vi "Get Function Status.vi"(8 "error in (no error)":errorcluster, 10 "Function.lvclass":refnum<class "Function.lvclass">, 11 "Results in":refnum<class "Results.lvclass">) -> (0 "error out":errorcluster, 3 "Results out":refnum<class "Results.lvclass">)   [LabVIEW 2016, in "Result Actor.lvlib" / "Results.lvclass"]
uses:
  <userlib>/Common Components/Results/Results.lvclass
  <userlib>/Common Components/Function Actor/Function.lvclass
  <userlib>/Common Components/Controller/Unique Function ID.ctl
  <userlib>/Common Components/Function Actor/Function.lvclass/Function.ctl
  <userlib>/Common Components/Results/Results.lvclass/Results.ctl
  <userlib>/Common Components/Controller/Controller.lvclass
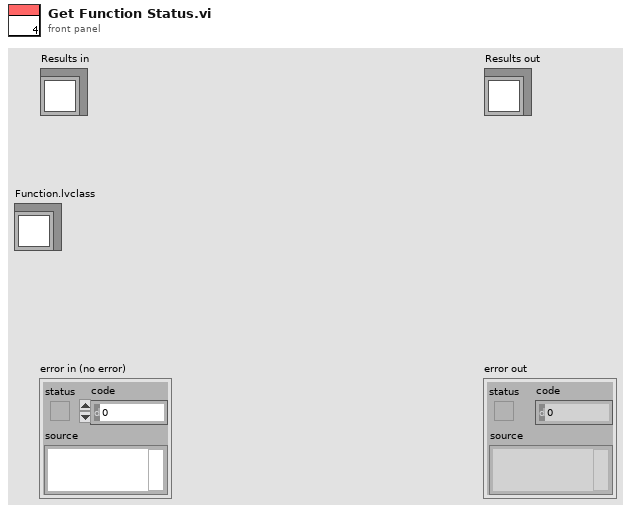
[diagram p1: front panel]
types:
  T1 = typedef "Controller Actor.lvlib/Controller.lvclass/Unique Function ID.ctl" = cluster{"Function Name":string, "Device Names":string[]}
  T2 = cluster{"Function Name":string, "Device Names":string[], "Time Stamp":timestamp}
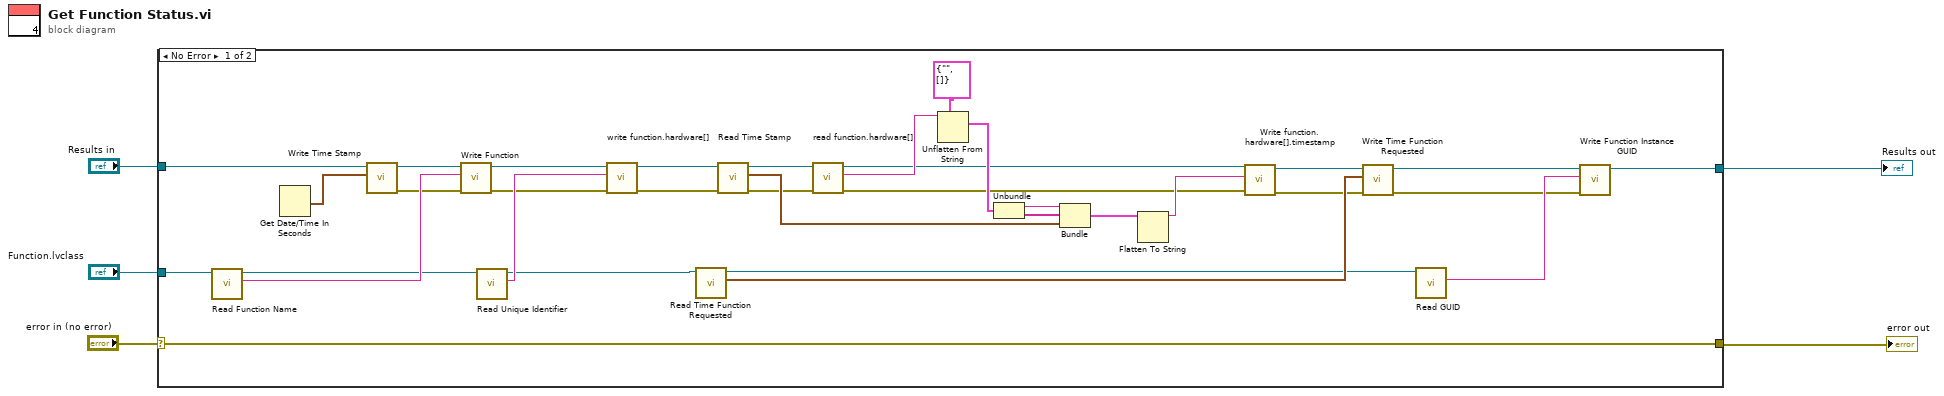
[diagram p0: block diagram]
diagram:
  n1 = case shown="No Error" "error in (no error)" {
    selector: "error in (no error)" -> [w39 w41]
    tunnel: [w39 w41] -> w4
    tunnel: [w14 w40] -> w2
    tunnel: "Results in" -> [w36 w40]
    tunnel: "Function.lvclass" -> [w34 _]
    frame No Error {
      n2 = call <userlib>:"Read Function Name.vi"("Function in"=w34) -> ("Function Name"=w35:string, "Function out"=w32:refnum<class "Function.lvclass">)  [unwired: 8 in, 1 out]
      n3 = Get Date/Time In Seconds() -> (seconds since 1Jan1904=w38:timestamp)
      n4 = call <userlib>:"Write Time Stamp.vi"("Time Stamp"=w38, "Results in"=w36) -> ("error out"=w12:errorcluster, "Results out"=w37:refnum<class "Results.lvclass">)  [unwired: 8 in]
      n5 = call <userlib>:"Write Function.vi"("error in (no error)"=w12, "Function"=w35, "Results in"=w37) -> ("error out"=w11:errorcluster, "Results out"=w33:refnum<class "Results.lvclass">)  [unwired: 7 in]
      n6 = call <userlib>:"Read Unique Identifier.vi"("Function in"=w32) -> ("Unique Identifier"=w31:string, "Function out"=w17:refnum<class "Function.lvclass">)  [unwired: 8 in, 1 out]
      n7 = call <userlib>:"write function.hardware[].vi"("error in (no error)"=w11, "uniqueid"=w31, "Results in"=w33) -> ("error out"=w10:errorcluster, "Results out"=w22:refnum<class "Results.lvclass">)  [unwired: 7 in]
      n8 = call <userlib>:"Read Time Function Requested.vi"("Function in"=w17) -> ("Time Function Requested"=w16:timestamp, "Function out"=w15:refnum<class "Function.lvclass">)  [unwired: 8 in, 1 out]
      n9 = call <userlib>:"Read Time Stamp.vi"("error in (no error)"=w10, "Results in"=w22) -> ("error out"=w9:errorcluster, "Time Stamp"=w30:timestamp, "Results out"=w28:refnum<class "Results.lvclass">)  [unwired: 7 in]
      n10 = call <userlib>:"read function.hardware[].vi"("error in (no error)"=w9, "Results in"=w28) -> ("error out"=w8:errorcluster, "uniqueid"=w23:string, "Results out"=w20:refnum<class "Results.lvclass">)  [unwired: 7 in]
      n11 = Unflatten From String(type=T1 {"Function Name"="", "Device Names"=[]} ("output cluster"), binary string=w23) -> (value=w26:T1)  [unwired: 3 in, 2 out]
      n12 = Unbundle(w26) -> ("Function Name"=w25:string, "Device Names"=w24:string[])
      n13 = Bundle("Function Name"=w25, "Device Names"=w24, "Time Stamp"=w30) -> (w29:T2)  [unwired: 1 in]
      n14 = Flatten To String(anything=w29) -> (data string=w21:string)  [unwired: 3 in, 2 out]
      n15 = call <userlib>:"Write function.hardware[].timestamp.vi"("error in (no error)"=w8, "function.hardware[].timestamp"=w21, "Results in"=w20) -> ("error out"=w7:errorcluster, "Results out"=w19:refnum<class "Results.lvclass">)  [unwired: 7 in]
      n16 = call <userlib>:"Write Time Function Requested.vi"("error in (no error)"=w7, "Time Function Requested"=w16, "Results in"=w19) -> ("error out"=w6:errorcluster, "Results out"=w18:refnum<class "Results.lvclass">)  [unwired: 7 in]
      n17 = call <userlib>:"Read GUID.vi"("Function in"=w15) -> ("GUID"=w13:string)  [unwired: 8 in, 2 out]
      n18 = call <userlib>:"Write Function Instance GUID.vi"("error in (no error)"=w6, "Function Instance GUID"=w13, "Results in"=w18) -> ("Results out"=w14:refnum<class "Results.lvclass">)  [unwired: 7 in, 1 out]
    }
    frame Error {
    }
  }
  "error out" <- w4
  "Results out" <- w2
